vi "State9-Exit.vi"(11 "Numeric":dbl) -> (1 "Cluster":T2, 2 "Front/Back 2":enum16{"Forward", "Backward", "Stop"}(ring), 3 "Left/Right":enum16{"Left", "Right", "Stop"}(ring), 4 "f":T1, 5 "Left/Right Speed":u32)   [LabVIEW 2014]
uses:
  FPGA Bitfiles/Parking States Indicators.ctl
  FPGA Bitfiles/Parking States.ctl
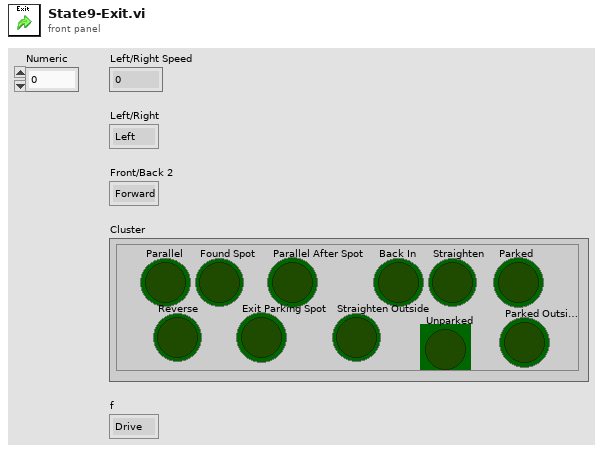
[diagram p1: front panel]
types:
  T1 = typedef "Parking States.ctl" = enum16{"Drive", "Parallel", "Found Spot", "Parallel After Spot", "Back In", "Straighten", "Parked", "Reverse", "Exit Parking Spot", "Straighten Outside", "Unparked", "Parked Outside"}
  T2 = typedef "Parking States Indicators.ctl" = cluster{"Parallel":bool, "Found Spot":bool, "Parallel After Spot":bool, "Back In":bool, "Straighten":bool, "Parked":bool, "Reverse":bool, "Exit Parking Spot":bool, "Straighten Outside":bool, "Unparked":bool, "Parked Outside":bool}
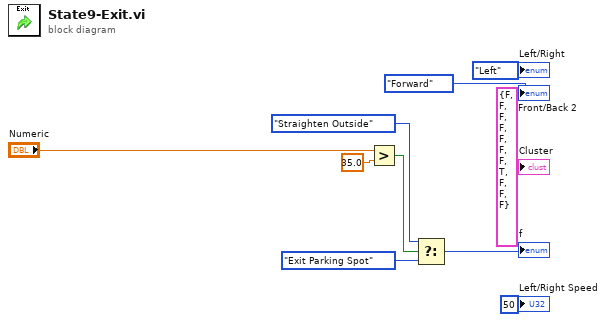
[diagram p0: block diagram]
diagram:
  n1 = Greater?(x="Numeric", y=35.0) -> (0:w5:bool)
  n2 = Select(t=Parking_States."Straighten Outside", s=w5, f=Parking_States."Exit Parking Spot") -> (s? t:f=→"f":T1)
  "Cluster" <- T2 {"Parallel"=FALSE, "Found Spot"=FALSE, "Parallel After Spot"=FALSE, "Back In"=FALSE, "Straighten"=FALSE, "Parked"=FALSE, "Reverse"=FALSE, "Exit Parking Spot"=TRUE, "Straighten Outside"=FALSE, "Unparked"=FALSE, "Parked Outside"=FALSE} ("Cluster")
  "Front/Back 2" <- enum16{"Forward", "Backward", "Stop"}."Forward" ("Front/Back 2")
  "Left/Right" <- enum16{"Left", "Right", "Stop"}."Left" ("Left/Right")
  "Left/Right Speed" <- u32 50 ("Left/Right Speed")
